vi "Advanced Connection Settings Polymporhic.vi"(6 "Advanced Connection Settings Cluster In":T1 caption="Advanced Connection Settings Cluster" {"Flow Control" items=["None", "XON/XOFF", "RTS/CTS", "XON/XOFF & RTS/CTS", "DTR/DSR", "XON/XOFF & DTR/DSR"]; "Stop Bits" items=["1.0"=10, "1.5"=15, "2.0"=20]; "Parity" items=["None", "Odd", "Even", "Mark", "Space"]; "Baud Rate" items=["100"=100, "300"=300, "600"=600, "1200"=1200, "2400"=2400, "4800"=4800, "9600"=9600, "14400"=14400, "19200"=1920, "28800"=28800, "38400"=38400, "56000"=56000, "57600"=57600, "115200"=13]}, 8 "error in (no error)":errorcluster, 10 "XML Elements":string) -> (0 "error out":errorcluster, 1 "Advanced Connection Settings Cluster Out":T1 caption="Advanced Connection Settings Cluster" {"Flow Control" items=["None", "XON/XOFF", "RTS/CTS", "XON/XOFF & RTS/CTS", "DTR/DSR", "XON/XOFF & DTR/DSR"]; "Stop Bits" items=["1.0"=10, "1.5"=15, "2.0"=20]; "Parity" items=["None", "Odd", "Even", "Mark", "Space"]; "Baud Rate" items=["100"=100, "300"=300, "600"=600, "1200"=1200, "2400"=2400, "4800"=4800, "9600"=9600, "14400"=14400, "19200"=1920, "28800"=28800, "38400"=38400, "56000"=56000, "57600"=57600, "115200"=13]})   [LabVIEW 2014]
uses:
  Controls/Advanced Connection Settings Cluster.ctl
panel:
  # "ADVANCED CONNECTION SETTINGS"
  # "ADVANCED CONNECTION SETTINGS"
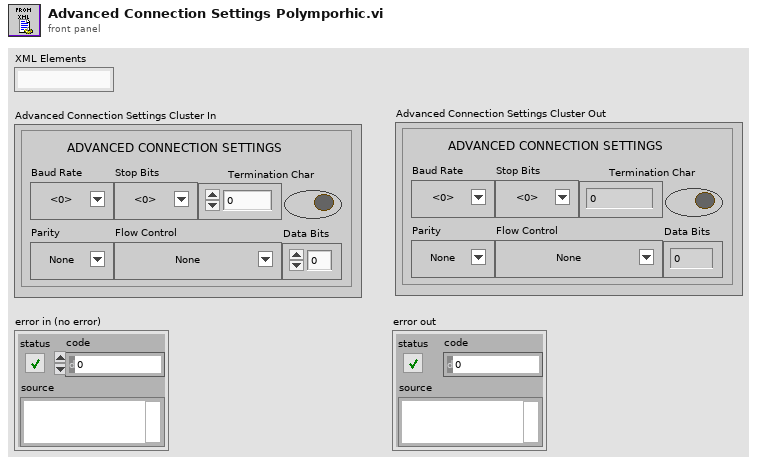
[diagram p1: front panel]
types:
  T1 = typedef "Advanced Connection Settings Cluster.ctl" = cluster{"Baud Rate":u32, "Data Bits":u16, "Parity":u16, "Stop Bits":u16, "Flow Control":u16, "Termination Char":u8, "Enable Termination Char":bool}
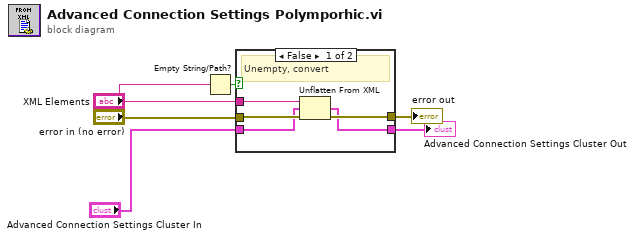
[diagram p0: block diagram]
diagram:
  n1 = Empty String/Path?(string/path="XML Elements") -> (empty?=w1:bool)
  n2 = case shown="False" w1 {
    tunnel: "error in (no error)" -> [w11 w12]
    tunnel: "Advanced Connection Settings Cluster In" -> [w8 w13]
    tunnel: [w7 w13] -> w4
    tunnel: [w10 w12] -> w5
    tunnel: "XML Elements" -> [w9 _]
    frame False {
      # "Unempty, convert"
      n3 = Unflatten From XML(xml string=w9, type=w8, error in (no error)=w11) -> (value=w7:T1, error out=w10:errorcluster)
    }
    frame True {
      # "Empty, default values"
    }
  }
  "error out" <- w5
  "Advanced Connection Settings Cluster Out" <- w4
